vi "PSK_init.vi"(9 "filter parameters":T3={"Alpha"=0.5, "Filter Length"=6, "TX Filter"=enum."Root Raised Cos"} {"Alpha" format="%.2f"}, 10 "QPSK System Parameters":T4={"Samples per Symbol"=8, "symbol map"=[], "Differential PSK"=enum."disable", "PSK type"=0, "M-PSK (4)"=4} {"PSK type" items=["normal", "shifted", "offset"]; "symbol map" format="%.3f"}) -> (0 "pulse shaping filter coefficients":dbl[](array[numeric]) format="%.2f", 1 "PSK synchronization parameters":T2 {"sync sequence" format="%.2f"}, 2 "matched filter coefficients":dbl[](array[numeric]) format="%.2f", 3 "PSK system parameters":T1 {"PSK type" items=["normal", "shifted", "offset"]; "symbol map" format="%.3f"})   [LabVIEW 2014]
uses:
  <vilib>/addons/Modulation/Digital/General/MT Generate Bits (Galois, PN Order).vi
  <vilib>/addons/Modulation/Digital/Support/Common/Validators/mod_Generate Bits Validate.vi
  <vilib>/addons/Modulation/Analog/support/mod_Set Error Source.vi
  <vilib>/addons/Modulation/Digital/General/MT Generate PSK System Parameters(M).vi
  <vilib>/addons/Modulation/Digital/Support/Common/Validators/mod_Generate Filter Coefficients Validate.vi
  <vilib>/addons/Modulation/Digital/General/subVIs/mod_Generate Filter Coefficients.vi
  <vilib>/addons/Modulation/Digital/General/subVIs/mod_Generate Bits PN Sequence.vi
  <vilib>/addons/Modulation/Digital/General/MT Generate PSK Synchronization Parameters (bit array).vi
  <vilib>/addons/Modulation/niDMT.lvlib
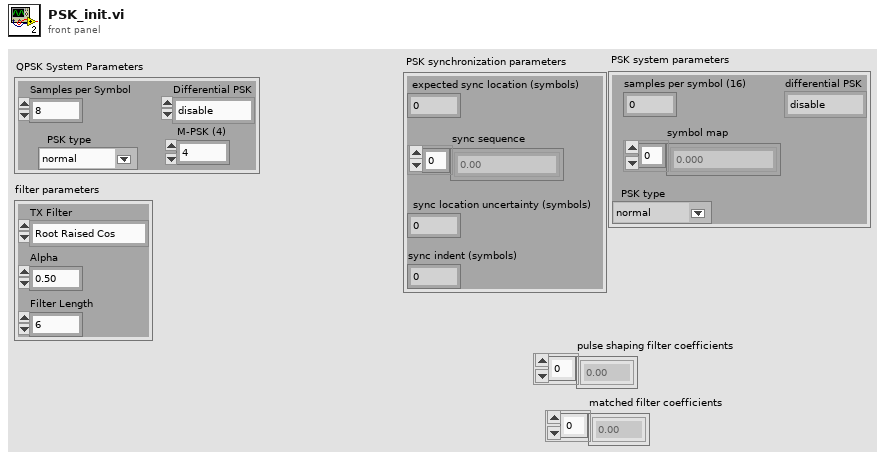
[diagram p1: front panel]
types:
  T1 = cluster{"samples per symbol (16)":i32, "symbol map":cdb[], "differential PSK":enum16{"disable", "enable"}, "PSK type":u16}
  T2 = cluster{"expected sync location (symbols)":i32, "sync sequence":cdb[], "sync location uncertainty (symbols)":i32, "sync indent (symbols)":i32}
  T3 = cluster{"Alpha":dbl, "Filter Length":i32, "TX Filter":enum16{"none", "Raised Cosine", "Root Raised Cos", "Gaussian"}}
  T4 = cluster{"Samples per Symbol":i32, "symbol map":cdb[], "Differential PSK":enum16{"disable", "enable"}, "PSK type":u16, "M-PSK (4)":i32}
  T5 = enum16{"FSK", "PSK", "QAM", "MSK", "PAM", "ASK", "CPM"}
  T6 = enum16{"none", "Raised Cosine", "Root Raised Cos", "Gaussian"}
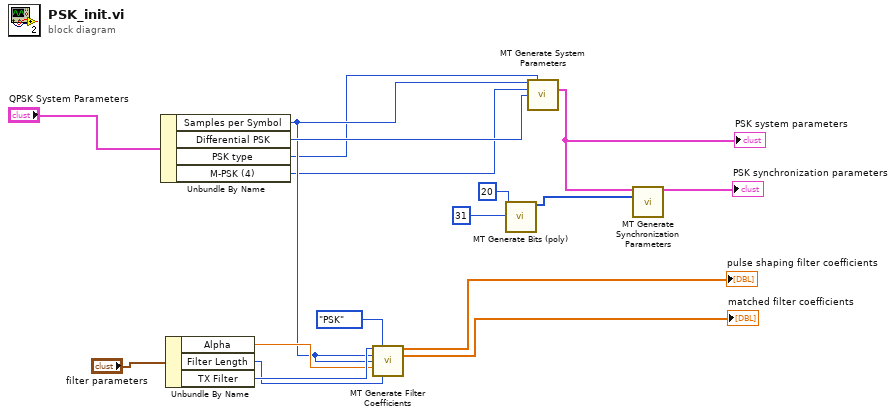
[diagram p0: block diagram]
diagram:
  n1 = Unbundle By Name("QPSK System Parameters") -> ("Samples per Symbol"=w8:i32, "Differential PSK"=w11:enum16{"disable", "enable"}, "PSK type"=w5:u16, "M-PSK (4)"=w4:i32)
  n2 = Unbundle By Name("filter parameters") -> ("Alpha"=w14:dbl, "Filter Length"=w15:i32, "TX Filter"=w16:T6)
  n3 = call <vilib>:"MT Generate Filter Coefficients.vi"("pulse shaping filter (none)"=w16, "modulation type"=T5."PSK", "pulse shaping samples per symbol (16)"=w8, "matched samples per symbol (16)"=w8, "filter parameter"=w14, "filter length (symbols)"=w15) -> ("pulse shaping filter coefficients"=→"pulse shaping filter coefficients":dbl[], "matched filter coefficients"=→"matched filter coefficients":dbl[])  [unwired: 7 in, 1 out]
  n4 = call-poly <vilib>:"MT Generate Bits (poly).vi"("total bits (128)"=20, "PN sequence order (9)"=31) -> ("output bit stream"=w7:i8[])  [unwired: 11 in, 2 out]
  n5 = call-poly <vilib>:"MT Generate System Parameters.vi"("samples per symbol (16)"=w8, "PSK type"=w5, "M-PSK (4)"=w4, "differential PSK"=w11) -> ("PSK system parameters"=w6:T1)  [unwired: 9 in, 2 out]
  "PSK system parameters" <- w6
  n6 = call-poly <vilib>:"MT Generate Synchronization Parameters.vi"("PSK system parameters"=w6, "sync bits"=w7) -> ("PSK synchronization parameters"=→"PSK synchronization parameters":T2)  [unwired: 12 in, 1 out]
